vi "GetConfigFilepath.vi"(8 "error in":errorcluster) -> (0 "error out":errorcluster, 3 "Test Manager config":path)   [LabVIEW 2013, in "Caraya.lvlib" / "Basic Test Manager.lvclass"]
uses:
  Basic Test Manager.lvclass
  <vilib>/Utility/sysdir.llb/System Directory Type.ctl
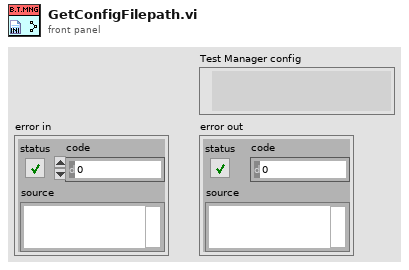
[diagram p1: front panel]
types:
  T1 = typedef "System Directory Type.ctl" = i32
  T2 = enum16{"open", "replace", "create", "open or create", "replace or create", "replace or create with confirmation"}
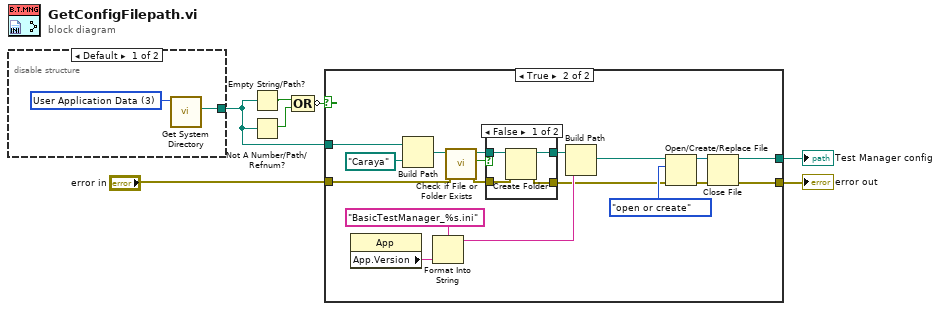
[diagram p0: block diagram]
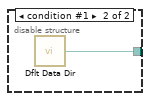
[diagram p2: hidden frame]
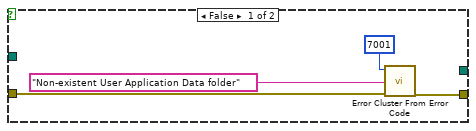
[diagram p3: hidden frame]
diagram:
  n1 = disable-structure shown="Default" {
    disable-tunnel: [w9 w10] -> w1
    frame condition #0 (active) {
      w8 = T1 3 items=["User Home"=0, "User Desktop"=1, "User Documents"=2, "User Application Data"=3, "User Preferences"=4, "User Temporary"=5, "Public Documents"=6, "Public Application Data"=7, "Public Preferences"=8, "Public Cache"=13, "System Core Libraries"=9, "System Installed Libraries"=10, "Application Files"=11, "Boot Volume Root"=12] ("system directory type")
      n2 = call <vilib>:"Get System Directory.vi"("system directory type"=w8) -> ("system directory"=w9:path)  [unwired: 10 in]
    }
    frame condition #1 {
      n3 = call <vilib>:"Dflt Data Dir.vi"() -> ("App:Default Data Directory"=w10:path)
    }
  }
  n4 = Empty String/Path?(string/path=w1) -> (empty?=w2:bool)
  n5 = Not A Number/Path/Refnum?(number/path/refnum=w1) -> (NaN/Path/Refnum?=w3:bool)
  n6 = Compound Arithmetic op=OR(w2, w3) -> (invert w4:bool)
  n7 = case shown="True" w4 {
    tunnel: w1 -> [_ w28]
    tunnel: [_ w26] -> w7
    tunnel: [w14 w22] -> w6
    tunnel: "error in" -> [w11 w18]
    frame False {
      n8 = call <vilib>:"Error Cluster From Error Code.vi"("error in (no error)"=w11, "error message (\"\")"="Non-existent User Application Data folder" ("error message (\"\")"), "error code (0)"=7001) -> ("error out"=w14:errorcluster)  [unwired: 6 in]
    }
    frame True {
      n9 = property class="App"() -> ("App.Version"=w31:string)  [unwired: 2 in, 2 out]
      n10 = Build Path(base path=w28, name or relative path=path "Caraya") -> (appended path=w20:path)
      n11 = Format Into String(format string="BasicTestManager_%s.ini", w31) -> (resulting string=w29:string)  [unwired: 2 in, 1 out]
      n12 = call <vilib>:"Check if File or Folder Exists.vi"("error in (no error)"=w18, "path"=w20) -> ("error out"=w17:errorcluster, "file or folder exists?"=w15:bool, "dup path"=w19:path)  [unwired: 7 in]
      n13 = case shown="False" w15 {
        tunnel: [w36 w38] -> w21
        tunnel: w19 -> [w35 w38]
        tunnel: w17 -> [w34 w37]
        tunnel: [w33 w37] -> w16
        frame False {
          n14 = Create Folder(path (use dialog)=w35, error in=w34) -> (created path=w36:path, error out=w33:errorcluster)  [unwired: 1 in, 1 out]
        }
        frame True {
        }
      }
      n15 = Build Path(base path=w21, name or relative path=w29) -> (appended path=w25:path)
      n16 = Open/Create/Replace File(file path (use dialog)=w25, error in=w16, operation (0:open)=T2."open or create") -> (refnum out=w27:refnum<file>, error out=w23:errorcluster)  [unwired: 3 in, 1 out]
      n17 = Close File(refnum=w27, error in=w23) -> (path=w26:path, error out=w22:errorcluster)
    }
  }
  "Test Manager config" <- w7
  "error out" <- w6
